vi "_Simulator PIM Tree.vi"   [LabVIEW 2011]
uses:
  PIM Command.ctl
panel:
  # "Simulator PIM Driver Tree\nSee Diagram"
types:
  T1 = typedef "PIM Command.ctl" = enum16{"LOAD", "KEEP ALIVE", "VALIDATE", "INITIALIZE", "PRESET", "GET CALIBRATION", "SET STIMULUS", "TOGGLE TX POWER", "SET TX ON", "SET TX OFF", "MEASURE", "UNLOAD"}
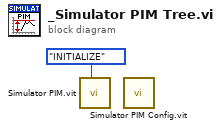
[diagram p0: block diagram]
diagram:
  n1 = call "Simulator PIM.vit"("PIM Command"=PIM_Command."INITIALIZE") -> ()  [unwired: 8 in, 3 out]
  n2 = call "Simulator PIM Config.vit"() -> ()  [unwired: 7 in, 5 out]
